vi "QueryServer_Invoke_GetRequest.vi"(6 "error in (no error)":errorcluster, 9 "gRPCid":T1) -> (0 "error out":errorcluster, 1 "parameter":string, 2 "command":string, 3 "gRPCid out":T1)   [LabVIEW 2019]
uses:
  QueryServer_gRPCid.ctl
  QueryServer_InvokeRequest.ctl
  Debug/labview_query_server.dll
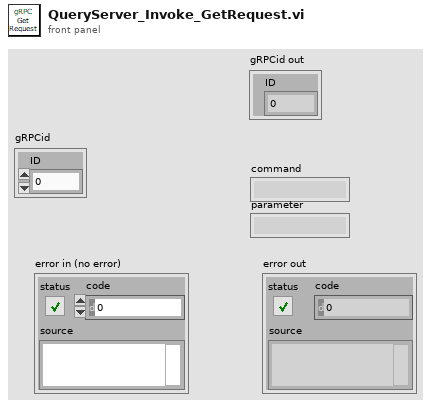
[diagram p1: front panel]
types:
  T1 = typedef "QueryServer_gRPCid.ctl" = cluster{"ID":u64}
  T2 = typedef "QueryServer_InvokeRequest.ctl" = cluster{"command":string, "parameter":string}
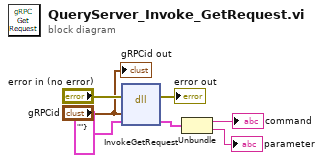
[diagram p0: block diagram]
diagram:
  n1 = dll-call lib="C:/dev/labview-grpc-query-server/Debug/labview_query_server.dll" fn="InvokeGetRequest"(error in="error in (no error)", "id"="gRPCid", "data"=T2 {"command"="", "parameter"=""} ("InvokeRequest")) -> (error out=→"error out":errorcluster, "data"=w3:T2)  [unwired: 4 in, 1 out]
  n2 = Unbundle(w3) -> ("command"=→"command":string, "parameter"=→"parameter":string)
  "gRPCid out" <- "gRPCid"
